vi "Engine Simulation 8 cylinder FPGA.vi"() -> ()   [LabVIEW 2014]
uses:
  <vilib>/NI/Engine Simulation Toolkit (EST)/Version Token.ctl
  <vilib>/NI/Engine Simulation Toolkit (EST)/APU/Settings.ctl
  <vilib>/NI/Engine Simulation Toolkit (EST)/APU/Input.ctl
  <vilib>/NI/Engine Simulation Toolkit (EST)/APU/Output.ctl
  <vilib>/NI/Engine Simulation Toolkit (EST)/Analog Replay/Settings.ctl
  <vilib>/NI/Engine Simulation Toolkit (EST)/Analog Replay/Input.ctl
  <vilib>/NI/Engine Simulation Toolkit (EST)/Analog Replay/Load Input.ctl
  <vilib>/NI/Engine Simulation Toolkit (EST)/Digital Pattern Generation/Load Input.ctl
  <vilib>/NI/Engine Simulation Toolkit (EST)/Digital Pattern Generation/Settings.ctl
  <vilib>/NI/Engine Simulation Toolkit (EST)/Digital Pattern Generation/Input.ctl
  <vilib>/NI/Engine Simulation Toolkit (EST)/ECU Event/Timing/Measure Output.ctl
  <vilib>/NI/Engine Simulation Toolkit (EST)/ECU Event/Timing/Measure Settings.ctl
  <vilib>/NI/Engine Simulation Toolkit (EST)/ECU Event/Timing/Capture Output.ctl
  <vilib>/NI/Engine Simulation Toolkit (EST)/Knock Sensor/Cylinder Input.ctl
  <vilib>/NI/Engine Simulation Toolkit (EST)/Knock Sensor/Cylinder Settings.ctl
  <vilib>/NI/Engine Simulation Toolkit (EST)/Knock Sensor/Generate Input.ctl
  <vilib>/NI/Engine Simulation Toolkit (EST)/Knock Sensor/Generate Settings.ctl
  <vilib>/NI/Engine Simulation Toolkit (EST)/Directional Speed/Load Input.ctl
  <vilib>/NI/Engine Simulation Toolkit (EST)/Directional Speed/Settings.ctl
  <vilib>/NI/Engine Simulation Toolkit (EST)/Directional Speed/Input.ctl
  <vilib>/NI/Engine Simulation Toolkit (EST)/APU/Shared Settings.ctl
  <vilib>/Platform/TimedLoop/XDataNode/timing_clust.ctl
  <vilib>/Platform/TimedLoop/XDataNode/nitl_modes.ctl
  <vilib>/Platform/TimedLoop/XDataNode/wakeup.ctl
  <vilib>/NI/Engine Simulation Toolkit (EST)/ECU Event/Timing/Capture Settings.ctl
  <vilib>/rvi/Emulation/niFpgaGetClockAttributes.vi
  <vilib>/rvi/Emulation/niFpgaSctlEmulationGetInTimedLoop.vi
  <vilib>/rvi/Emulation/niFpgaEmulationReportErrorSimple.vi
  <vilib>/rvi/Emulation/niFpgaCriticalErrorInLSC.vi
  <vilib>/rvi/Emulation/niFpgaProcessEmulError.vi
  <vilib>/rvi/eio/common/nirviEmuTemplateMethod_errors.vi
  <vilib>/rvi/DataTransferAndStorage/Container/Common/niFpgaContainerGetUniqueNameForEmu.vi
  <vilib>/rvi/DataTransferAndStorage/Container/Common/niFpgaContainerSetEmuInfo.vi
  <vilib>/rvi/eio/common/nirviEmuReportErrorAndStop.vi
  <vilib>/NI/Engine Simulation Toolkit (EST)/ECU Event/Timing/Measure Events (40MHz).vi
  <vilib>/Platform/TimedLoop/XDataNode/XDataNode.xnode
  <vilib>/eio/EIONode/EIONode.xnode
  <vilib>/rvi/LocalResourceManager/LocalResourceManager.xnode
  <vilib>/Platform/TimedLoop/XDataNode/XDNodeRunTimeDep.lvlib
  <userlib>/_NI VeriStand FPGA Support/NI VeriStand FPGA Clock Support/NI_VS FPGA Clock Support.lvlib
  <vilib>/NI Veristand/FPGA/NI_VS FPGA Support.lvlib
  <vilib>/NI/Engine Simulation Toolkit (EST)/APU/APU.lvlib
  <vilib>/NI/Engine Simulation Toolkit (EST)/Analog Replay/Analog Replay.lvlib
  <vilib>/NI/Engine Simulation Toolkit (EST)/Digital Pattern Generation/Digital Pattern Generation.lvlib
  <vilib>/NI/Engine Simulation Toolkit (EST)/ECU Event/Timing/ECU Event Timing.lvlib
  <vilib>/NI/Engine Simulation Toolkit (EST)/Knock Sensor/Knock Sensor.lvlib
  <vilib>/NI/Engine Simulation Toolkit (EST)/Directional Speed/Directional Speed.lvlib
  <vilib>/NI/Engine Simulation Toolkit (EST)/Engine Simulation Toolkit.lvlib
panel:
  in  "Tab Control":T1(tab)
  in  "Start":bool
  in  "Loop Rate (usec)":u32
  in  "Write to  RTSI":bool
  in  "Use External Timing":bool
  in  "Generate IRQ":bool
  in  "shared settings.apu 1":T2 {"start" format="%#.15g"}
  in  "go.apu 1":bool
  in  "settings.apu 1":T3 caption="settings"
  out "output.apu 1":T4 caption="output"
  in  "input.apu 1":T5={"desired speed"=0.0, "reset"=TRUE} caption="input"
  in  "est.version":T6
  in  "Spark Tics to Filter":fxp<+,11,11>=350.0
  out "status.Event Spark 6":T7
  out "status.Event Spark 5":T7
  out "status.Event Spark 4":T7
  out "status.Event Spark 3":T7
  out "status.Event Spark 2":T7
  out "status.Event Spark 1":T7
  in  "settings.Event Spark 6":T8
  in  "settings.Event Spark 5":T8
  in  "settings.Event Spark 4":T8
  in  "settings.Event Spark 3":T8
  in  "settings.Event Spark 2":T8
  in  "settings.Event Spark 1":T8
  out "capture.Event Spark 6.Event 1":T9
  out "capture.Event Spark 5.Event 1":T9
  out "capture.Event Spark 4.Event 1":T9
  out "capture.Event Spark 3.Event 1":T9
  out "capture.Event Spark 2.Event 1":T9
  out "capture.Event Spark 1.Event 1":T9
  out "status.Event Spark 7":T7
  in  "settings.Event Spark 7":T8
  out "capture.Event Spark 7.Event 1":T9
  out "status.Event Spark 8":T7
  in  "settings.Event Spark 8":T8
  out "capture.Event Spark 8.Event 1":T9
  in  "Inj Tics to Filter":fxp<+,11,11>=100.0
  out "status.Event Inj 1":T7
  in  "settings.Event Inj 1":T8
  out "capture.Event Inj 1.Event 1":T9
  out "capture.Event Inj 1.Event 2":T9
  out "capture.Event Inj 1.Event 3":T9
  out "capture.Event Inj 1.Event 4":T9
  out "capture.Event Inj 1.Event 5":T9
  out "capture.Event Inj 2.Event 4":T9
  out "capture.Event Inj 2.Event 3":T9
  out "capture.Event Inj 2.Event 2":T9
  out "status.Event Inj 2":T7
  in  "settings.Event Inj 2":T8
  out "capture.Event Inj 2.Event 1":T9
  out "capture.Event Inj 2.Event 5":T9
  out "capture.Event Inj 3.Event 5":T9
  out "capture.Event Inj 3.Event 4":T9
  out "capture.Event Inj 3.Event 3":T9
  out "capture.Event Inj 3.Event 2":T9
  out "status.Event Inj 3":T7
  in  "settings.Event Inj 3":T8
  out "capture.Event Inj 3.Event 1":T9
  out "capture.Event Inj 4.Event 3":T9
  out "capture.Event Inj 4.Event 2":T9
  out "status.Event Inj 4":T7
  in  "settings.Event Inj 4":T8
  out "capture.Event Inj 4.Event 1":T9
  out "capture.Event Inj 4.Event 4":T9
  out "capture.Event Inj 4.Event 5":T9
  in  "settings.Event Inj 7":T8
  in  "settings.Event Inj 6":T8
  in  "settings.Event Inj 8":T8
  in  "settings.Event Inj 5":T8
  out "status.Event Inj 5":T7
  out "capture.Event Inj 5.Event 1":T9
  out "capture.Event Inj 5.Event 5":T9
  out "status.Event Inj 8":T7
  out "capture.Event Inj 8.Event 5":T9
  out "capture.Event Inj 6.Event 3":T9
  out "capture.Event Inj 6.Event 2":T9
  out "status.Event Inj 7":T7
  out "capture.Event Inj 8.Event 4":T9
  out "capture.Event Inj 8.Event 3":T9
  out "capture.Event Inj 8.Event 2":T9
  out "capture.Event Inj 8.Event 1":T9
  out "status.Event Inj 6":T7
  out "capture.Event Inj 6.Event 1":T9
  out "capture.Event Inj 5.Event 4":T9
  out "capture.Event Inj 5.Event 3":T9
  out "capture.Event Inj 5.Event 2":T9
  out "capture.Event Inj 6.Event 5":T9
  out "capture.Event Inj 6.Event 4":T9
  out "capture.Event Inj 7.Event 5":T9
  out "capture.Event Inj 7.Event 4":T9
  out "capture.Event Inj 7.Event 3":T9
  out "capture.Event Inj 7.Event 2":T9
  out "capture.Event Inj 7.Event 1":T9
  in  "load input.Dir Speed 1":T10
  in  "settings.Dir Speed 2":T11
  in  "input.Dir Speed 2":T12
  in  "settings.Dir Speed 1":T11
  in  "input.Dir Speed 1":T12
  in  "load input.Dir Speed 2":T10
  in  "load input.Crank":T13
  in  "settings.Aux Pattern":T14
  in  "input.Aux Pattern":T15
  in  "settings.Cam 2":T14
  in  "input.Cam 2":T15
  in  "settings.Cam 1":T14
  in  "input.Cam 1":T15
  in  "settings.Crank":T14
  in  "input.Crank":T15
  in  "load input.Cam 1":T13
  in  "load input.Cam 2":T13
  in  "load input.Aux Pattern":T13
  in  "settings.VR 1":T16 caption="settings"
  in  "settings.VR 2":T16 caption="settings"
  in  "input.VR 2":T17 caption="input"
  in  "input.VR 1":T17 caption="input"
  in  "load input.VR 1":T18={"Data"=[0, 0, 0, 0, 0, 0, 0, 0, 0, 0, 0, 0, 0, 0, 0, 0], "LoadOffset"=0, "Done"=FALSE} caption="input"
  in  "load input.VR 2":T18={"Data"=[0, 0, 0, 0, 0, 0, 0, 0, 0, 0, 0, 0, 0, 0, 0, 0], "LoadOffset"=0, "Done"=FALSE} caption="input"
  in  "input.Knock 1.Cylinder 4":T19={"probability compare"=65535, "high freq scaler"=0.0, "trigger position"=0}
  in  "input.Knock 1.Cylinder 3":T19={"probability compare"=65535, "high freq scaler"=0.0, "trigger position"=0}
  in  "input.Knock 1.Cylinder 2":T19={"probability compare"=65535, "high freq scaler"=0.0, "trigger position"=0}
  in  "input.Knock 1.Cylinder 1":T19={"probability compare"=65535, "high freq scaler"=0.0, "trigger position"=0}
  in  "settings.Knock 1.Cylinder 4":T20
  in  "settings.Knock 1.Cylinder 3":T20
  in  "settings.Knock 1.Cylinder 2":T20
  in  "settings.Knock 1.Cylinder 1":T20
  in  "input.Knock 1":T21
  in  "settings.Knock 1":T22
  in  "input.Knock 1.Cylinder 5":T19={"probability compare"=65535, "high freq scaler"=0.0, "trigger position"=0}
  in  "settings.Knock 1.Cylinder 5":T20
  in  "input.Knock 1.Cylinder 8":T19={"probability compare"=65535, "high freq scaler"=0.0, "trigger position"=0}
  in  "settings.Knock 1.Cylinder 8":T20
  in  "input.Knock 1.Cylinder 7":T19={"probability compare"=65535, "high freq scaler"=0.0, "trigger position"=0}
  in  "settings.Knock 1.Cylinder 7":T20
  in  "input.Knock 1.Cylinder 6":T19={"probability compare"=65535, "high freq scaler"=0.0, "trigger position"=0}
  in  "settings.Knock 1.Cylinder 6":T20
  in  "input.Knock 2.Cylinder 4":T19
  in  "input.Knock 2.Cylinder 3":T19
  in  "input.Knock 2.Cylinder 2":T19
  in  "input.Knock 2.Cylinder 1":T19
  in  "settings.Knock 2.Cylinder 4":T20
  in  "settings.Knock 2.Cylinder 3":T20
  in  "settings.Knock 2.Cylinder 2":T20
  in  "settings.Knock 2.Cylinder 1":T20
  in  "input.Knock 2.Cylinder 7":T19
  in  "settings.Knock 2.Cylinder 7":T20
  in  "input.Knock 2.Cylinder 5":T19
  in  "settings.Knock 2.Cylinder 5":T20
  in  "input.Knock 2.Cylinder 8":T19
  in  "settings.Knock 2.Cylinder 8":T20
  in  "input.Knock 2.Cylinder 6":T19
  in  "settings.Knock 2.Cylinder 6":T20
  in  "input.Knock 2":T21
  in  "settings.Knock 2":T22
  in  "PulseGen Packets 0-7":u64[](array[numeric])=[0, 0, 0, 0, 0, 0, 0, 0]
  in  "PWM.In.7.Timeout":u32=40000
  in  "PWM.In.6.Timeout":u32=40000
  in  "PWM.In.5.Timeout":u32=40000
  in  "PWM.In.4.Timeout":u32=40000
  in  "PWM.In.3.Timeout":u32=40000
  in  "PWM.In.2.Timeout":u32=40000
  in  "PWM.In.1.Timeout":u32=40000
  in  "PWM.In.0.Timeout":u32=40000
  out "PulseMeas Packets 0-7":u64[](array[numeric])
  in  "PWM.In.15.Timeout":u32=40000
  in  "PWM.In.14.Timeout":u32=40000
  in  "PWM.In.13.Timeout":u32=40000
  in  "PWM.In.12.Timeout":u32=40000
  in  "PWM.In.11.Timeout":u32=40000
  in  "PWM.In.10.Timeout":u32=40000
  in  "PWM.In.9.Timeout":u32=40000
  in  "PWM.In.8.Timeout":u32=40000
  out "PulseMeas Packets 2 8-15":u64[](array[numeric])
  in  "PulseGen Packets 8-15":u64[](array[numeric])=[0, 0, 0, 0, 0, 0, 0, 0]
  in  "PulseMeas 7 Timeout":u32=40000
  in  "PulseMeas 6 Timeout":u32=40000
  in  "PulseMeas 5 Timeout":u32=40000
  in  "PulseMeas 4 Timeout":u32=40000
  in  "PulseMeas 3 Timeout":u32=40000
  in  "PulseMeas 2 Timeout":u32=40000
  in  "PulseMeas 1 Timeout":u32=40000
  in  "PulseMeas 0 Timeout":u32=40000
  out "PulseMeas Packets 8-15":u64[](array[numeric])
  in  "PulseGen Packets":u64[](array[numeric])=[0, 0, 0, 0, 0, 0, 0, 0]
  # "DC"
  # "f"
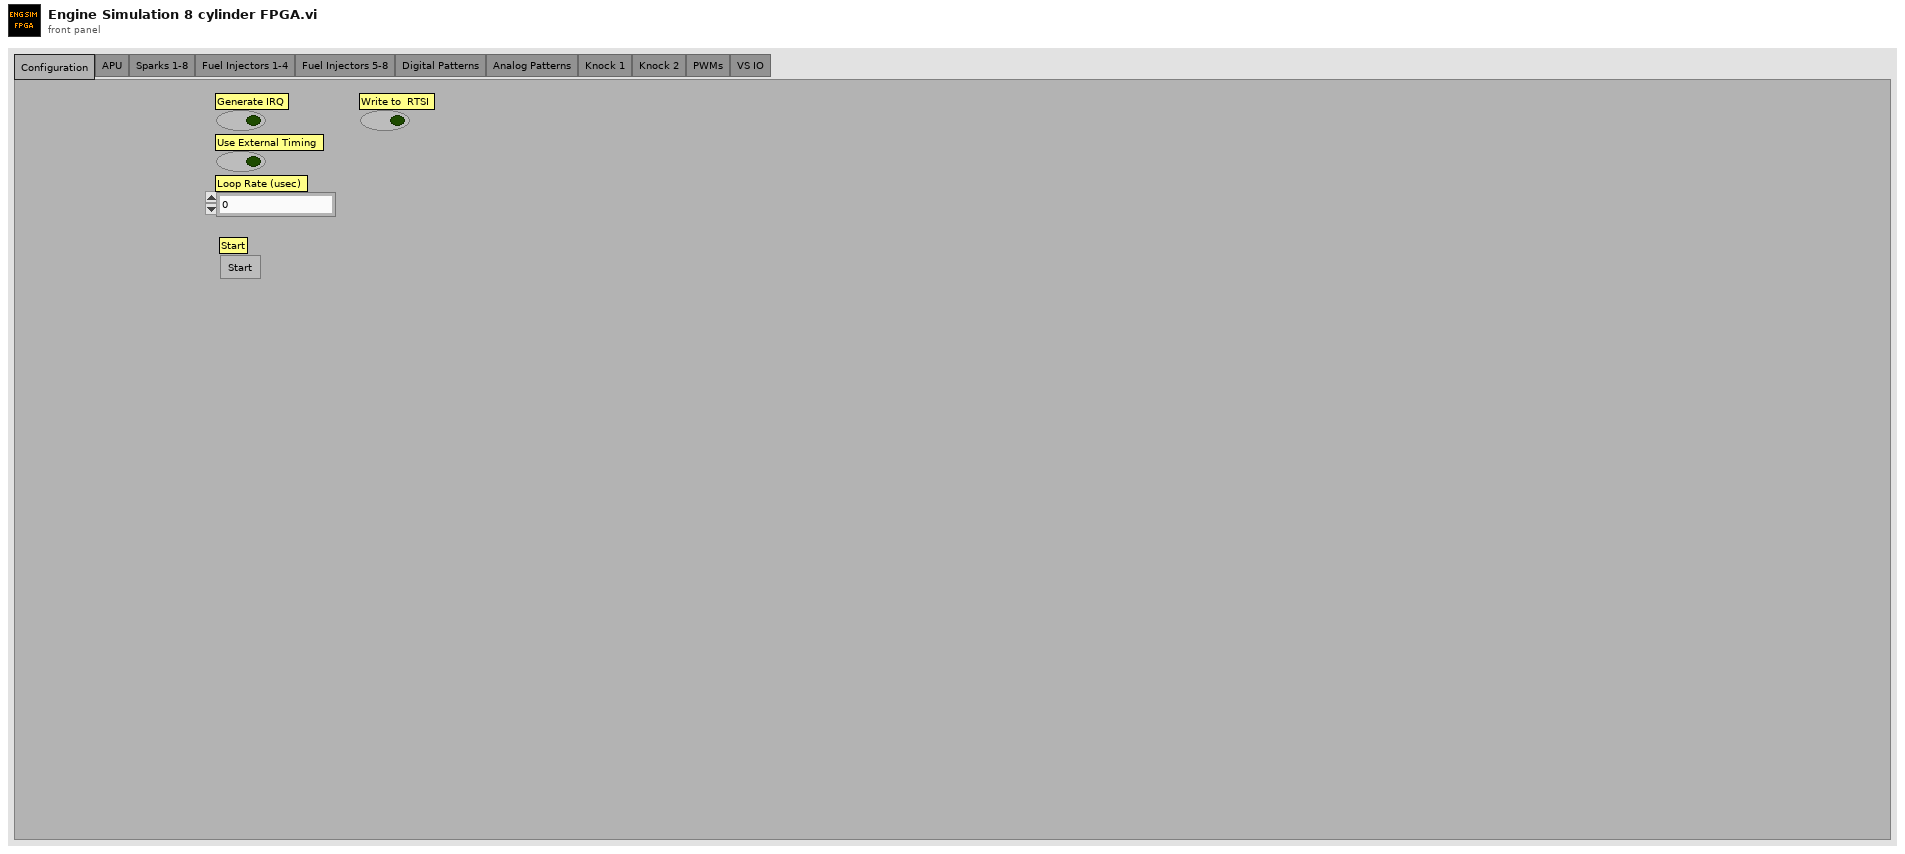
[diagram p1: front panel]
types:
  T1 = enum32{"Configuration", "APU", "Sparks 1-8", "Fuel Injectors 1-4", "Fuel Injectors 5-8", "Digital Patterns", "Analog Patterns", "Knock 1", "Knock 2", "PWMs", "VS IO"}
  T2 = typedef "Engine Simulation Toolkit.lvlib/APU.lvlib/Shared Settings.ctl" = cluster{"start":fxp<+,17,17>, "stuck limit":fxp<+,18,18>}
  T3 = typedef "Engine Simulation Toolkit.lvlib/APU.lvlib/Settings.ctl" = cluster{"acceleration":fxp<+,18,-20>, "enable accel":bool}
  T4 = typedef "Engine Simulation Toolkit.lvlib/APU.lvlib/Output.ctl" = cluster{"crank":u16, "cycle":u16, "actual speed":fxp<+/-,23,2>}
  T5 = typedef "Engine Simulation Toolkit.lvlib/APU.lvlib/Input.ctl" = cluster{"desired speed":fxp<+/-,23,2>, "reset":bool}
  T6 = typedef "Engine Simulation Toolkit.lvlib/Version Token.ctl" = cluster{"1.3.0":bool}
  T7 = typedef "Engine Simulation Toolkit.lvlib/ECU Event Timing.lvlib/Measure Output.ctl" = cluster{"stuck active":bool, "window all active":bool, "window orphan start":bool, "window orphan end":bool}
  T8 = typedef "Engine Simulation Toolkit.lvlib/ECU Event Timing.lvlib/Measure Settings.ctl" = cluster{"max":u16, "min":u16, "active high":bool, "wrap":bool}
  T9 = typedef "Engine Simulation Toolkit.lvlib/ECU Event Timing.lvlib/Capture Output.ctl" = cluster{"Start":u16, "End":u16, "Duration (tics)":fxp<+,18,18>, "Event present":bool}
  T10 = typedef "Engine Simulation Toolkit.lvlib/Directional Speed.lvlib/Load Input.ctl" = cluster{"address":fxp<+,10,10>, "done":bool, "angle":u16}
  T11 = typedef "Engine Simulation Toolkit.lvlib/Directional Speed.lvlib/Settings.ctl" = cluster{"Upper Value":u16, "Lower Value":u16, "Upper Index":fxp<+,10,10>, "Lower Index":fxp<+,10,10>, "Enabled":bool}
  T12 = typedef "Engine Simulation Toolkit.lvlib/Directional Speed.lvlib/Input.ctl" = cluster{"td (tics)":u16, "tf (tics)":u16, "tr (tics)":u16}
  T13 = typedef "Engine Simulation Toolkit.lvlib/Digital Pattern Generation.lvlib/Load Input.ctl" = cluster{"address":fxp<+,11,11>, "done":bool, "angle":u16}
  T14 = typedef "Engine Simulation Toolkit.lvlib/Digital Pattern Generation.lvlib/Settings.ctl" = cluster{"edge 1":u16, "edge 2":u16, "cycle angle":bool, "enabled":bool, "first falling":bool, "fault":bool, "fault wrap":bool, "fault value":bool, "fault count":fxp<+,4,4>, "use fault count":bool}
  T15 = typedef "Engine Simulation Toolkit.lvlib/Digital Pattern Generation.lvlib/Input.ctl" = cluster{"Offset":i16}
  T16 = typedef "Engine Simulation Toolkit.lvlib/Analog Replay.lvlib/Settings.ctl" = cluster{"ReverseNegate":bool, "CycleAngle":bool, "SpeedThreshold":fxp<+/-,23,2>, "AOBelowThreshold":i16}
  T17 = typedef "Engine Simulation Toolkit.lvlib/Analog Replay.lvlib/Input.ctl" = cluster{"Offset":i16, "VScaleSlope":fxp<+,18,6>, "VScaleIntercept":fxp<+/-,18,3>}
  T18 = typedef "Engine Simulation Toolkit.lvlib/Analog Replay.lvlib/Load Input.ctl" = cluster{"Data":i16[], "LoadOffset":u16, "Done":bool}
  T19 = typedef "Engine Simulation Toolkit.lvlib/Knock Sensor.lvlib/Cylinder Input.ctl" = cluster{"probability compare":u16, "high freq scaler":fxp<+,10,0>, "trigger position":u16}
  T20 = typedef "Engine Simulation Toolkit.lvlib/Knock Sensor.lvlib/Cylinder Settings.ctl" = cluster{"seed":u16, "reset":bool}
  T21 = typedef "Engine Simulation Toolkit.lvlib/Knock Sensor.lvlib/Generate Input.ctl" = cluster{"low freq scaler":fxp<+,10,0>}
  T22 = typedef "Engine Simulation Toolkit.lvlib/Knock Sensor.lvlib/Generate Settings.ctl" = cluster{"low freq (periods/tick)":fxp<+,32,0>, "high freq (periods/tick)":fxp<+,32,0>, "duration (1.25MHz tics)":fxp<+,18,18>, "low freq speed slope":fxp<+,16,-3>, "low freq speed intercept":fxp<+,10,-10>, "low freq by speed":bool}
  T23 = typedef "XDNodeRunTimeDep.lvlib/timing_clust.ctl" = cluster{"Expected End [f-1]":u64, "Actual End [f-1]":u64, "Finished Late? [f-1]":bool, "Expected End [i-1]":u64, "Actual End [i-1]":u64, "Finished Late? [i-1]":bool, "Expected Start [i]":u64, "Actual Start [i]":u64, "Expected Start [f]":u64, "Actual Start [f]":u64, "Source Name":string, "Structure Name":string, "Period":i64, "Deadline":i64, "Offset":i64, "Start":i64, "Priority":i32, "Timeout":i32, "Mode":T24, "Wakeup Reason":T25, "Error":errorcluster, "Source Type":string, "Secondary Source Type":string, "Global End Time":u64, "Global Start Time":u64, "Frame Duration":u64, "Iteration Duration":u64, "Assigned CPU":i32, "I/O Scan Engine Mode":u32}
  T24 = typedef "XDNodeRunTimeDep.lvlib/nitl_modes.ctl" = enum32{"No Change", "Process missed periods, maintain original phase", "Discard missed periods, maintain original phase", "Process missed periods, ignore original phase", "Discard missed periods, ignore original phase"}
  T25 = typedef "XDNodeRunTimeDep.lvlib/wakeup.ctl" = enum32{"Normal", "Aborted", "Asynchronous wakeup", "Timing source error", "Timed loop error", "Timeout"}
  T26 = cluster{"DO0":refnum<k21>, "DO1":refnum<k21>, "DO2":refnum<k21>, "DO3":refnum<k21>, "DO4":refnum<k21>, "DO5":refnum<k21>, "DO6":refnum<k21>, "DO7":refnum<k21>}
  T27 = cluster{"DI0":refnum<k21>, "DI1":refnum<k21>, "DI2":refnum<k21>, "DI3":refnum<k21>, "DI4":refnum<k21>, "DI5":refnum<k21>, "DI6":refnum<k21>, "DI7":refnum<k21>}
  T28 = typedef "Engine Simulation Toolkit.lvlib/Digital Pattern Generation.lvlib/Load Data.ctl" = cluster{"max address":fxp<+,11,11>, "memory":refnum<k21>}
  T29 = typedef "Engine Simulation Toolkit.lvlib/APU.lvlib/Register Bus.ctl" = cluster{"Speed":refnum<k21>, "Crank Angle":refnum<k21>, "Cycle Angle":refnum<k21>, "Crank Count":refnum<k21>, "Cycle Count":refnum<k21>, "1.25 MHz Counter":refnum<k21>, "Crank Rollover":refnum<k21>, "Cycle Rollover":refnum<k21>, "shared settings":T2}
  T30 = typedef "Engine Simulation Toolkit.lvlib/Directional Speed.lvlib/Load Data.ctl" = cluster{"max address":fxp<+,10,10>, "Memory":refnum<k21>}
  T31 = typedef "Engine Simulation Toolkit.lvlib/Knock Sensor.lvlib/Triggered Cylinder Data.ctl" = cluster{"trigger knock":bool, "high freq scaler":fxp<+,10,0>}
  T32 = typedef "Engine Simulation Toolkit.lvlib/ECU Event Timing.lvlib/Capture Settings.ctl" = u8
  T33 = typedef "Engine Simulation Toolkit.lvlib/ECU Event Timing.lvlib/Measured Data.ctl" = cluster{"start":u16, "end":u16, "duration (tics)":fxp<+,18,18>, "window end":bool, "window begin":bool, "pulse end":bool, "pulse #":u8}
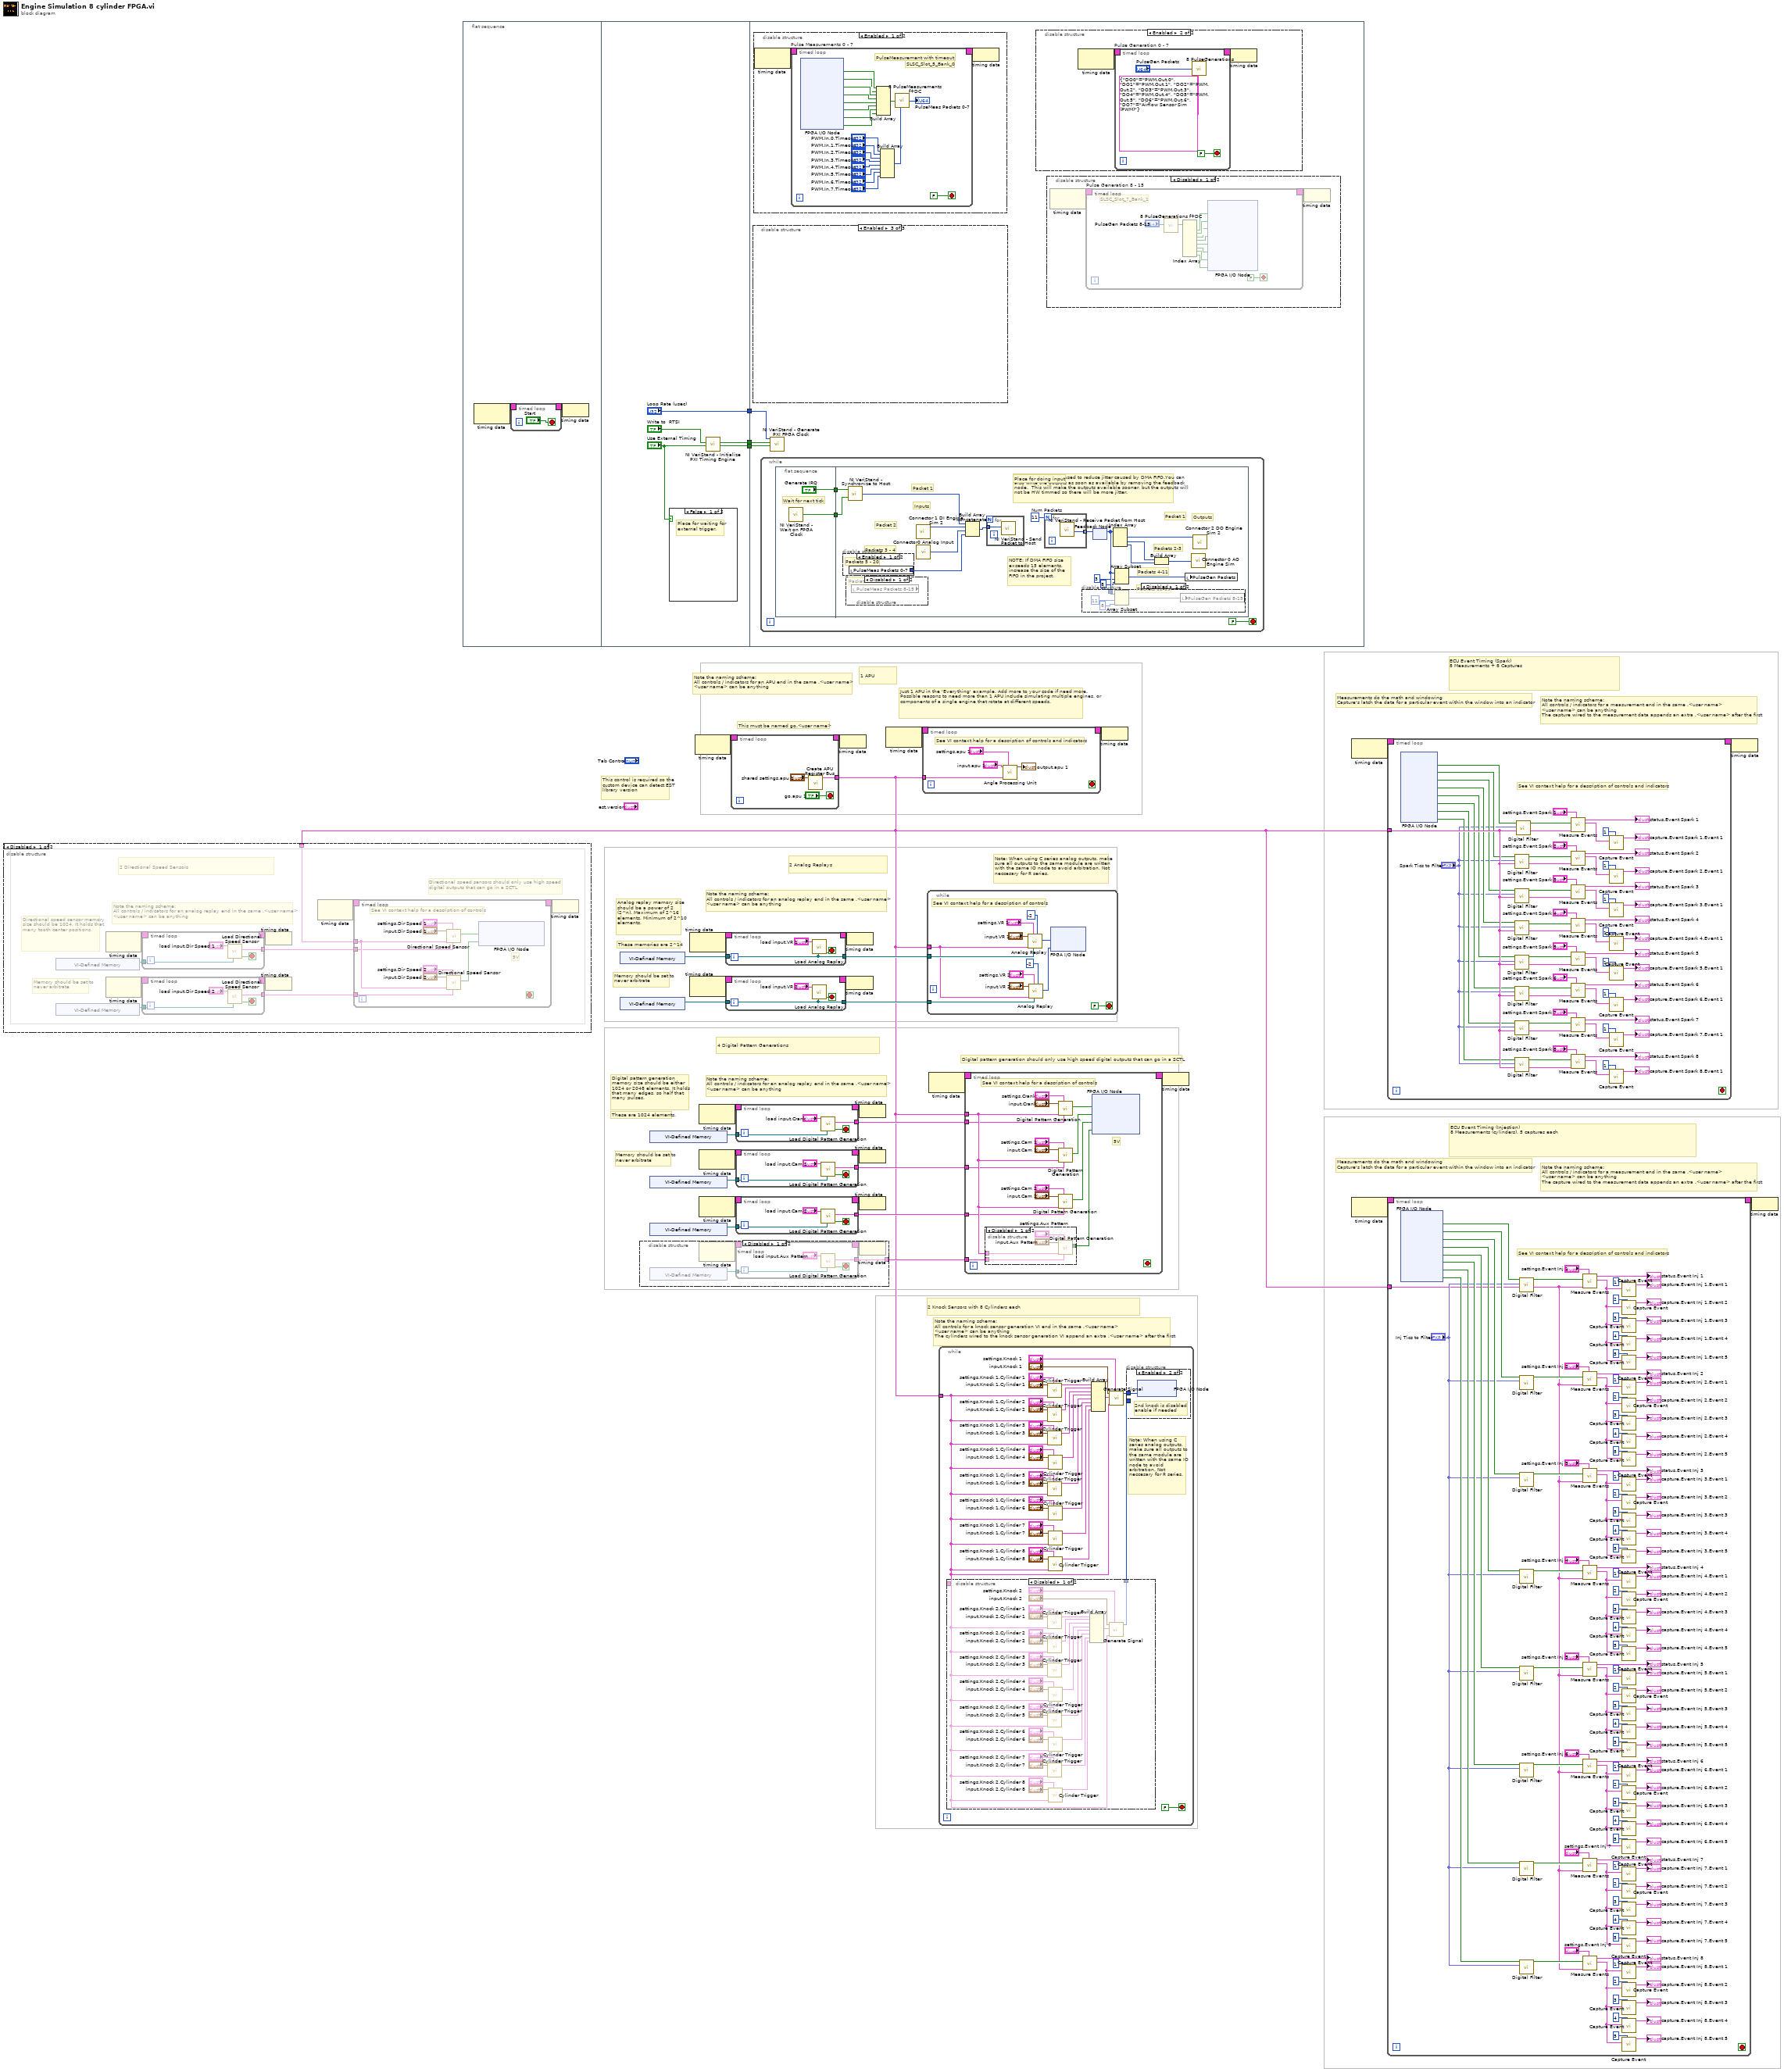
[diagram p0: block diagram]
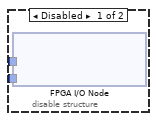
[diagram p5: hidden frame]
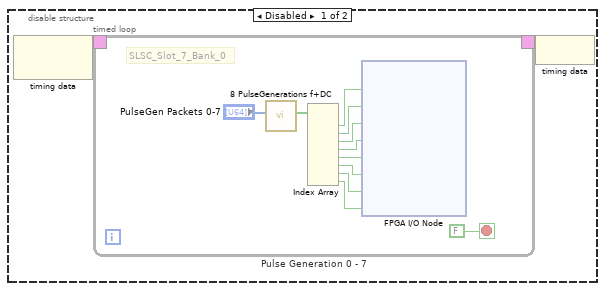
[diagram p9: hidden frame]
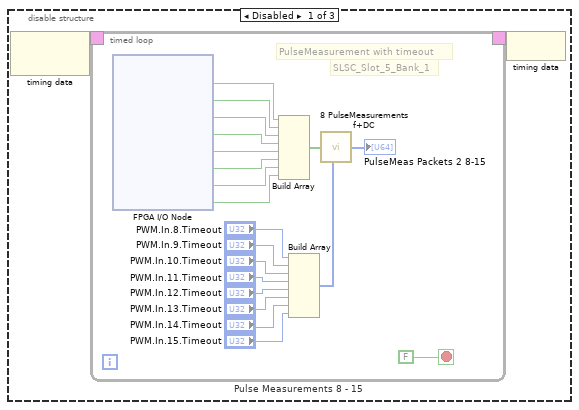
[diagram p11: hidden frame]
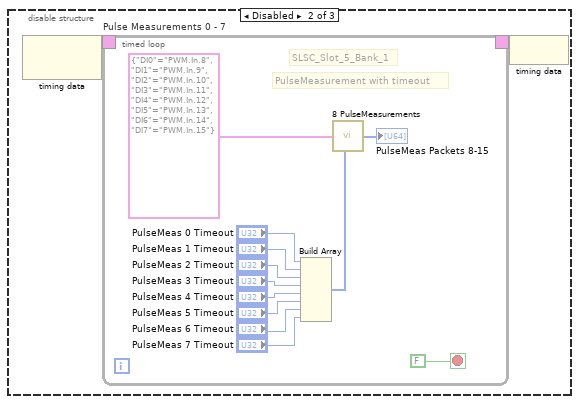
[diagram p12: hidden frame]
diagram:
  # "This must be named go.<user name>"
  # "Memory should be set to never arbitrate"
  # "Memory should be set to never arbitrate"
  # "Note the naming scheme: \nAll controls for a knock sensor generation VI end in the same .<user name>\n<user name> can be anything\nThe cylinders wired to the knock sensor generation VI append an extra .<user name> after the first"
  # "2 Knock Sensors with 8 Cylinders each"
  # "Measurements do the math and windowing\nCapture's latch the data for a particular event within the window into an indicator"
  # "ECU Event Timing (Injection)\n8 Measurements (cylinders), 5 captures each"
  # "Note the naming scheme: \nAll controls / indicators for a measurement end in the same .<user name>\n<user name> can be anything\nThe capture wired to the measurement data appends an extra .<user name> after the first"
  # "Measurements do the math and windowing\nCapture's latch the data for a particular event within the window into an indicator"
  # "ECU Event Timing (Spark)\n8 Measurements + 8 Captures"
  # "Note the naming scheme: \nAll controls / indicators for a measurement end in the same .<user name>\n<user name> can be anything\nThe capture wired to the measurement data appends an extra .<user name> after the first"
  # "Digital pattern generation should only use high speed digital outputs that can go in a SCTL"
  # "4 Digital Pattern Generations"
  # "Note the naming scheme: \nAll controls / indicators for an analog replay end in the same .<user name>\n<user name> can be anything"
  # "These are 1024 elements."
  # "Digital pattern generation memory size should be either 1024 or 2048 elements. It holds that many edges, so half that many pulses."
  # "Note: When using C series analog outputs, make sure all outputs to the same module are written with the same IO node to avoid arbitration. Not neccesary for R series."
  # "2 Analog Replays"
  # "1 APU"
  # "These memories are 2^14"
  # "Note the naming scheme: \nAll controls / indicators for an APU end in the same .<user name>\n<user name> can be anything"
  # "Note the naming scheme: \nAll controls / indicators for an analog replay end in the same .<user name>\n<user name> can be anything"
  # "Analog replay memory size should be a power of 2 (2^n). Maximum of 2^16 elements. Minimum of 2^10 elements."
  # "Just 1 APU in the 'Everything' example. Add more to your code if need more. Possible reasons to need more than 1 APU include simulating multiple engines, or components of a single engine that rotate at different speeds."
  # "This control is required so the custom device can detect EST library version"
  n1 = flat-sequence {
    tunnel: [w44] -> w35
    tunnel: ["Loop Rate (usec)"] -> w34
    tunnel: [w43] -> w33
    tunnel: w35 -> [w50]
    tunnel: w34 -> [w49]
    tunnel: w33 -> [w48]
    frame #0 {
      n2 = node-c288() -> (w37:T23)  [unwired: 1 out]
      n3 = timed-loop {
        timing: w37 -> [_]
        timing-out: [_] -> w36
        stop <- "Start" stop-if-true
      }
      n4 = node-c288(w36) -> ()
    }
    frame #1 {
      n5 = case shown="False" "Use External Timing" {
        frame False {
          # "Place for waiting for external trigger."
        }
        frame True {
          # "Do not wait on trigger when externally timed."
        }
      }
      n6 = call <userlib>:"NI VeriStand - Initialize PXI Timing Engine.vi"("Use External Timing In"="Use External Timing", "Write to  RTSI In"="Write to  RTSI") -> ("Use External Timing Out"=w44:bool, "Write to  RTSI Out"=w43:bool)  [unwired: 8 in]
    }
    frame #2 {
      n7 = disable-structure shown="Enabled" {
        frame Disabled {
          n8 = node-c288() -> (w121:T23)  [unwired: 1 out]
          n9 = timed-loop "Pulse Measurements 8 - 15" {
            timing: w121 -> [_]
            timing-out: [_] -> w120
            stop <- FALSE stop-if-true
            # "SLSC_Slot_5_Bank_1"
            # "PulseMeasurement with timeout"
            n10 = xnode "FPGA I/O Node"() -> ("PWM.In.8"=w124:bool, "PWM.In.9"=w125:bool, "PWM.In.10"=w126:bool, "PWM.In.11"=w127:bool, "PWM.In.12"=w128:bool, "PWM.In.13"=w129:bool, "PWM.In.14"=w130:bool, "PWM.In.15"=w123:bool)  [unwired: 8 in, 8 out]
            n11 = Build Array(w124, w125, w126, w127, w128, w129, w130, w123) -> (w122:bool[])
            n12 = Build Array("PWM.In.8.Timeout", "PWM.In.9.Timeout", "PWM.In.10.Timeout", "PWM.In.11.Timeout", "PWM.In.12.Timeout", "PWM.In.13.Timeout", "PWM.In.14.Timeout", "PWM.In.15.Timeout") -> (w140:u32[])
            n13 = call "8 PulseMeasurements f+DC.vi"("8 PulseMeas Chs"=w122, "PulseMeas Timeouts"=w140) -> ("PulseMeas Packets DC-f"=→"PulseMeas Packets 2 8-15":u64[])  [unwired: 7 in]
          }
          n14 = node-c288(w120) -> ()
        }
        frame Disabled {
          n15 = node-c288() -> (w147:T23)  [unwired: 1 out]
          n16 = timed-loop "Pulse Measurements 0 - 7" {
            timing: w147 -> [_]
            timing-out: [_] -> w146
            stop <- FALSE stop-if-true
            # "SLSC_Slot_5_Bank_1"
            # "PulseMeasurement with timeout"
            n17 = Build Array("PulseMeas 0 Timeout", "PulseMeas 1 Timeout", "PulseMeas 2 Timeout", "PulseMeas 3 Timeout", "PulseMeas 4 Timeout", "PulseMeas 5 Timeout", "PulseMeas 6 Timeout", "PulseMeas 7 Timeout") -> (w158:u32[])
            n18 = call <userlib>:"8 PulseMeasurements.vi"("8 PulseMeas Chs"=T27 {"DI0"="PWM.In.8", "DI1"="PWM.In.9", "DI2"="PWM.In.10", "DI3"="PWM.In.11", "DI4"="PWM.In.12", "DI5"="PWM.In.13", "DI6"="PWM.In.14", "DI7"="PWM.In.15"}, "PulseMeas Timeouts"=w158) -> ("PulseMeas Packets"=→"PulseMeas Packets 8-15":u64[])  [unwired: 7 in]
          }
          n19 = node-c288(w146) -> ()
        }
        frame Enabled {
        }
      }
      n20 = disable-structure shown="Enabled" {
        frame Enabled {
          n21 = node-c288() -> (w52:T23)  [unwired: 1 out]
          n22 = timed-loop "Pulse Measurements 0 - 7" {
            timing: w52 -> [_]
            timing-out: [_] -> w51
            stop <- FALSE stop-if-true
            # "SLSC_Slot_5_Bank_0"
            # "PulseMeasurement with timeout"
            n23 = xnode "FPGA I/O Node"() -> ("PWM.In.0"=w55:bool, "PWM.In.1"=w56:bool, "PWM.In.2"=w57:bool, "PWM.In.3"=w58:bool, "PWM.In.4"=w59:bool, "PWM.In.5"=w60:bool, "PWM.In.6"=w61:bool, "PWM.In.7"=w54:bool)  [unwired: 8 in, 8 out]
            n24 = Build Array(w55, w56, w57, w58, w59, w60, w61, w54) -> (w53:bool[])
            n25 = Build Array("PWM.In.0.Timeout", "PWM.In.1.Timeout", "PWM.In.2.Timeout", "PWM.In.3.Timeout", "PWM.In.4.Timeout", "PWM.In.5.Timeout", "PWM.In.6.Timeout", "PWM.In.7.Timeout") -> (w71:u32[])
            n26 = call "8 PulseMeasurements f+DC.vi"("8 PulseMeas Chs"=w53, "PulseMeas Timeouts"=w71) -> ("PulseMeas Packets DC-f"=→"PulseMeas Packets 0-7":u64[])  [unwired: 7 in]
          }
          n27 = node-c288(w51) -> ()
        }
        frame Disabled {
        }
      }
      n28 = while {
        stop <- FALSE stop-if-true
        n29 = flat-sequence {
          tunnel: ["Generate IRQ"] -> w165
          tunnel: [w167] -> w164
          tunnel: w165 -> [w185]
          tunnel: w164 -> [w184]
          frame #0 {
            # "Wait for next tick"
            n30 = call <userlib>:"NI VeriStand - Wait on FPGA Clock.vi"() -> ("Clock Ticked"=w167:bool)
          }
          frame #1 {
            w183 = 11  # Num Packets
            # "Packet 2"
            # "Packets 12-19"
            # "Packets 4-11"
            # "Packets 2-3"
            # "Packet 1"
            # "Packets 3 - 4"
            # "Inputs"
            # "Outputs"
            # "Packet 1"
            # "NOTE: If DMA FIFO size exceeds 15 elements, increase the size of the FIFO in the project."
            # "Feedback nodes are used to reduce jitter caused by DMA FIFO.You can also write the outputs as soon as available by removing the feedback node.  This will make the outputs available sooner, but the outputs will not be HW timmed so there will be more jitter."
            # "Place for doing input"
            n31 = disable-structure shown="Enabled" {
              disable-tunnel: [w186 _] -> w169
              frame Enabled {
                # "Packets 5 - 20"
                n32 = local read "PulseMeas Packets 0-7"() -> (w186:u64[])
              }
              frame Disabled {
              }
            }
            n33 = disable-structure shown="Disabled" {
              frame Disabled {
                # "Packets 21 - 28"
                n34 = local read "PulseMeas Packets 8-15"() -> ()  [unwired: 1 out]
              }
              frame Enabled {
              }
            }
            n35 = call <userlib>:"NI VeriStand - Synchronize to Host.vi"("Clock Ticked"=w184, "Generate IRQ"=w185) -> ("Is Late?"=w182:u64)
            n36 = call "Connector 1 DI Engine Sim 2.vi"() -> ("Packet"=w174:u64)  [unwired: 11 in]
            n37 = call <userlib>:"Connector0 Analog Input.vi"() -> ("Packets"=w180:u64[])
            n38 = Build Array (concatenate)(w182, w174, w180, w169) -> (w181:u64[])
            n39 = for {
              tunnel: w181 -> [w191] mode=indexing
              n40 = call <vilib>:"NI VeriStand - Send Packet to Host.vi"("Element"=w191) -> ()  [unwired: 2 in, 9 out]
            }
            n41 = for {
              N: w183 -> [_]
              tunnel: [w192] -> w179 mode=indexing
              n42 = call <vilib>:"NI VeriStand - Receive Packet from Host.vi"() -> ("Element"=w192:u64)  [unwired: 2 in, 9 out]
            }
            n43 = feedback-in #1(w179) -> ()
            n44 = feedback #1() -> (w173:u64[])  [unwired: 1 in]
            n45 = disable-structure shown="Disabled" {
              disable-tunnel: w173 -> [w190 _]
              frame Disabled {
                n46 = Array Subset(array=w190, index=11, length=8) -> (w187:u64[])
                n47 = local write "PulseGen Packets 8-15"(w187) -> ()
              }
              frame Enabled {
              }
            }
            n48 = Index Array(array=w173) -> (element #1=w175:u64, element #2=w178:u64, element #3=w177:u64)  [unwired: 3 in]
            n49 = Array Subset(array=w173, index=3, length=8) -> (w170:u64[])
            n50 = Build Array(w178, w177) -> (w176:u64[])
            n51 = local write "PulseGen Packets"(w170) -> ()
            n52 = call "Connector 0 AO Engine Sim.vi"("Packets"=w176) -> ()
            n53 = call "Connector 2 DO Engine Sim 2.vi"("Packet"=w175) -> ()  [unwired: 11 in]
          }
        }
      }
      n54 = call <userlib>:"NI VeriStand - Generate PXI FPGA Clock.vi"("Use External Timing"=w50, "Write to  RTSI"=w48, "Loop Rate (usec)"=w49) -> ()  [unwired: 9 in]
      n55 = disable-structure shown="Enabled" {
        frame Disabled {
          n56 = node-c288() -> (w78:T23)  [unwired: 1 out]
          n57 = timed-loop "Pulse Generation 0 - 7" {
            timing: w78 -> [_]
            timing-out: [_] -> w77
            stop <- FALSE stop-if-true
            # "SLSC_Slot_7_Bank_0"
            n58 = call "8 PulseGenerations f+DC.vi"("PulseGen Packets"="PulseGen Packets 0-7") -> ("PWMs"=w87:bool[])  [unwired: 8 in]
            n59 = Index Array(array=w87) -> (element #1=w86:bool, element #2=w85:bool, element #3=w84:bool, element #4=w83:bool, element #5=w82:bool, element #6=w81:bool, element #7=w80:bool, element #8=w79:bool)  [unwired: 8 in]
            n60 = xnode "FPGA I/O Node"("PWM.Out.0"=w86, "PWM.Out.1"=w85, "PWM.Out.2"=w84, "PWM.Out.3"=w83, "PWM.Out.4"=w82, "PWM.Out.5"=w81, "PWM.Out.6"=w80, "PWM.Out.7"=w79) -> ()  [unwired: 8 in, 8 out]
          }
          n61 = node-c288(w77) -> ()
        }
        frame Enabled {
          n62 = node-c288() -> (w95:T23)  [unwired: 1 out]
          n63 = timed-loop "Pulse Generation 0 - 7" {
            timing: w95 -> [_]
            timing-out: [_] -> w94
            stop <- FALSE stop-if-true
            n64 = call <userlib>:"8 PulseGenerations.vi"("PulseGen Packets"="PulseGen Packets", "8 PulseGen Chs"=T26 {"DO0"="PWM.Out.0", "DO1"="PWM.Out.1", "DO2"="PWM.Out.2", "DO3"="PWM.Out.3", "DO4"="PWM.Out.4", "DO5"="PWM.Out.5", "DO6"="PWM.Out.6", "DO7"="Airflow Sensor Sim (PWM)"}) -> ()  [unwired: 8 in]
          }
          n65 = node-c288(w94) -> ()
        }
      }
      n66 = disable-structure shown="Disabled" {
        frame Disabled {
          n67 = node-c288() -> (w104:T23)  [unwired: 1 out]
          n68 = timed-loop "Pulse Generation 8 - 15" {
            timing: w104 -> [_]
            timing-out: [_] -> w103
            stop <- FALSE stop-if-true
            # "SLSC_Slot_7_Bank_1"
            n69 = call "8 PulseGenerations f+DC.vi"("PulseGen Packets"="PulseGen Packets 8-15") -> ("PWMs"=w113:bool[])  [unwired: 8 in]
            n70 = Index Array(array=w113) -> (element #1=w112:bool, element #2=w111:bool, element #3=w110:bool, element #4=w109:bool, element #5=w108:bool, element #6=w107:bool, element #7=w106:bool, element #8=w105:bool)  [unwired: 8 in]
            n71 = xnode "FPGA I/O Node"("PWM.Out.8"=w112, "PWM.Out.9"=w111, "PWM.Out.10"=w110, "PWM.Out.11"=w109, "PWM.Out.12"=w108, "PWM.Out.13"=w107, "PWM.Out.14"=w106, "PWM.Out.15"=w105) -> ()  [unwired: 8 in, 8 out]
          }
          n72 = node-c288(w103) -> ()
        }
        frame Enabled {
        }
      }
    }
  }
  n73 = xnode "VI-Defined Memory"() -> ("Memory Out"=w11:refnum<k21>)
  n74 = xnode "VI-Defined Memory"() -> ("Memory Out"=w12:refnum<k21>)
  n75 = disable-structure shown="Disabled" {
    disable-tunnel: [w193 _] -> w4
    frame Disabled {
      n76 = xnode "VI-Defined Memory"() -> ("Memory Out"=w194:refnum<k21>)
      n77 = node-c288() -> (w196:T23)  [unwired: 1 in]
      n78 = timed-loop {
        timing: w196 -> [_]
        timing-out: [_] -> w195
        tunnel: w194 -> [w199]
        tunnel: [w198] -> w193
        stop <- w200 stop-if-true
        n79 = call <vilib>:"Load Digital Pattern Generation.vi"("memory"=w199, "load input.<user name>"="load input.Aux Pattern") -> ("done"=w200:bool, "load data"=w198:T28)  [unwired: 8 in]
      }
      n80 = node-c288(w195) -> ()
    }
    frame Enabled {
    }
  }
  n81 = xnode "VI-Defined Memory"() -> ("Memory Out"=w8:refnum<k21>)
  n82 = xnode "VI-Defined Memory"() -> ("Memory Out"=w6:refnum<k21>)
  n83 = xnode "VI-Defined Memory"() -> ("Memory Out"=w5:refnum<k21>)
  n84 = node-c288() -> (w30:T23)  [unwired: 1 in]
  n85 = node-c288() -> (w28:T23)  [unwired: 1 in]
  n86 = node-c288() -> (w14:T23)  [unwired: 1 in]
  n87 = node-c288() -> (w26:T23)  [unwired: 1 in]
  n88 = node-c288() -> (w22:T23)  [unwired: 1 in]
  n89 = node-c288() -> (w20:T23)  [unwired: 1 in]
  n90 = timed-loop {
    timing: w30 -> [_]
    timing-out: [_] -> w29
    tunnel: w11 -> [w205]
    tunnel: [w205] -> w10
    stop <- w206 stop-if-true
    n91 = call <vilib>:"Load Analog Replay.vi"("memory"=w205, "load input.<user name>"="load input.VR 1") -> ("done"=w206:bool)  [unwired: 9 in]
  }
  n92 = timed-loop {
    timing: w28 -> [_]
    timing-out: [_] -> w27
    tunnel: w12 -> [w210]
    tunnel: [w210] -> w9
    stop <- w211 stop-if-true
    n93 = call <vilib>:"Load Analog Replay.vi"("memory"=w210, "load input.<user name>"="load input.VR 2") -> ("done"=w211:bool)  [unwired: 9 in]
  }
  n94 = timed-loop {
    timing: w14 -> [_]
    timing-out: [_] -> w13
    tunnel: [w216] -> w1
    stop <- "go.apu 1" stop-if-true
    n95 = call <vilib>:"Create APU Register Bus.vi"("shared settings.<user name>"="shared settings.apu 1") -> ("register bus"=w216:T29)  [unwired: 10 in]
  }
  n96 = disable-structure shown="Disabled" {
    disable-tunnel: w1 -> [w220 _]
    frame Disabled {
      # "Memory should be set to never arbitrate"
      # "Note the naming scheme: \nAll controls / indicators for an analog replay end in the same .<user name>\n<user name> can be anything"
      # "Directional speed sensor memory size should be 1024. It holds that many tooth center positions."
      # "Directional speed sensors should only use high speed digital outputs that can go in a SCTL"
      # "2 Directional Speed Sensors"
      n97 = xnode "VI-Defined Memory"() -> ("Memory Out"=w221:refnum<k21>)
      n98 = xnode "VI-Defined Memory"() -> ("Memory Out"=w223:refnum<k21>)
      n99 = node-c288() -> (w230:T23)  [unwired: 1 in]
      n100 = node-c288() -> (w226:T23)  [unwired: 1 in]
      n101 = timed-loop {
        timing: w230 -> [_]
        timing-out: [_] -> w229
        tunnel: w221 -> [w254]
        tunnel: [w253] -> w222
        stop <- w255 stop-if-true
        n102 = call <vilib>:"Load Directional Speed Sensor.vi"("Memory In"=w254, "load input.<user name>"="load input.Dir Speed 1") -> ("done"=w255:bool, "load data"=w253:T30)  [unwired: 8 in]
      }
      n103 = timed-loop {
        timing: w226 -> [_]
        timing-out: [_] -> w225
        tunnel: w223 -> [w233]
        tunnel: [w232] -> w224
        stop <- w234 stop-if-true
        n104 = call <vilib>:"Load Directional Speed Sensor.vi"("Memory In"=w233, "load input.<user name>"="load input.Dir Speed 2") -> ("done"=w234:bool, "load data"=w232:T30)  [unwired: 8 in]
      }
      n105 = node-c288(w229) -> ()
      n106 = node-c288(w225) -> ()
      n107 = node-c288() -> (w228:T23)  [unwired: 1 in]
      n108 = timed-loop {
        tunnel: w220 -> [w241]
        timing: w228 -> [_]
        timing-out: [_] -> w227
        tunnel: w222 -> [w240]
        tunnel: w224 -> [w239]
        stop <- _ stop-if-true
        # "5V"
        # "See VI context help for a description of controls"
        n109 = call <vilib>:"Directional Speed Sensor.vi"("load data"=w240, "settings.<user name>"="settings.Dir Speed 1", "register bus"=w241, "input.<user name>"="input.Dir Speed 1") -> ("digial output"=w244:bool)  [unwired: 7 in]
        n110 = call <vilib>:"Directional Speed Sensor.vi"("load data"=w239, "settings.<user name>"="settings.Dir Speed 2", "register bus"=w241, "input.<user name>"="input.Dir Speed 2") -> ("digial output"=w245:bool)  [unwired: 7 in]
        n111 = xnode "FPGA I/O Node"("Directional Speed 1"=w244, "Directional Speed 2"=w245) -> ()  [unwired: 2 in, 2 out]
      }
      n112 = node-c288(w227) -> ()
    }
    frame Enabled {
    }
  }
  n113 = timed-loop {
    timing: w26 -> [_]
    timing-out: [_] -> w25
    tunnel: w8 -> [w262]
    tunnel: [w261] -> w7
    stop <- w263 stop-if-true
    n114 = call <vilib>:"Load Digital Pattern Generation.vi"("memory"=w262, "load input.<user name>"="load input.Crank") -> ("done"=w263:bool, "load data"=w261:T28)  [unwired: 8 in]
  }
  n115 = timed-loop {
    timing: w22 -> [_]
    timing-out: [_] -> w21
    tunnel: w6 -> [w268]
    tunnel: [w267] -> w2
    stop <- w269 stop-if-true
    n116 = call <vilib>:"Load Digital Pattern Generation.vi"("memory"=w268, "load input.<user name>"="load input.Cam 1") -> ("done"=w269:bool, "load data"=w267:T28)  [unwired: 8 in]
  }
  n117 = timed-loop {
    timing: w20 -> [_]
    timing-out: [_] -> w19
    tunnel: w5 -> [w274]
    tunnel: [w273] -> w3
    stop <- w275 stop-if-true
    n118 = call <vilib>:"Load Digital Pattern Generation.vi"("memory"=w274, "load input.<user name>"="load input.Cam 2") -> ("done"=w275:bool, "load data"=w273:T28)  [unwired: 8 in]
  }
  n119 = node-c288(w13) -> ()
  n120 = node-c288(w27) -> ()
  n121 = node-c288(w29) -> ()
  n122 = node-c288(w25) -> ()
  n123 = node-c288(w21) -> ()
  n124 = node-c288(w19) -> ()
  n125 = node-c288() -> (w32:T23)  [unwired: 1 in]
  n126 = timed-loop {
    timing: w32 -> [_]
    timing-out: [_] -> w31
    tunnel: w1 -> [w278]
    stop <- _ stop-if-true
    # "See VI context help for a description of controls and indicators"
    n127 = call <vilib>:"Angle Processing Unit.vi"("settings.<user name>"="settings.apu 1", "register bus"=w278, "input.<user name>"="input.apu 1") -> ("output.<user name>"=→"output.apu 1":T4)  [unwired: 8 in]
  }
  n128 = while {
    tunnel: w10 -> [w295]
    tunnel: w1 -> [w284]
    tunnel: w9 -> [w292]
    stop <- FALSE stop-if-true
    # "See VI context help for a description of controls"
    n129 = call <vilib>:"Analog Replay.vi"("shift"=i8 -2, "memory"=w295, "settings.<user name>"="settings.VR 1", "register bus"=w284, "input.<user name>"="input.VR 1") -> ("analog value"=w288:i16)  [unwired: 6 in]
    n130 = call <vilib>:"Analog Replay.vi"("shift"=i8 -2, "memory"=w292, "settings.<user name>"="settings.VR 2", "register bus"=w284, "input.<user name>"="input.VR 2") -> ("analog value"=w287:i16)  [unwired: 6 in]
    n131 = xnode "FPGA I/O Node"("VR 1"=w288, "VR 2"=w287) -> ()  [unwired: 2 in, 2 out]
  }
  n132 = node-c288() -> (w24:T23)  [unwired: 1 in]
  n133 = while {
    tunnel: w1 -> [w297]
    stop <- FALSE stop-if-true
    # "Note: When using C series analog outputs, make sure all outputs to the same module are written with the same IO node to avoid arbitration. Not neccesary for R series."
    n134 = disable-structure shown="Disabled" {
      disable-tunnel: w297 -> [w330 _]
      disable-tunnel: [w327 _] -> w296
      frame Disabled {
        n135 = call <vilib>:"Cylinder Trigger.vi"("settings.<user name>"="settings.Knock 2.Cylinder 1", "register bus"=w330, "input.<user name>"="input.Knock 2.Cylinder 1") -> ("triggered knock data"=w335:T31)  [unwired: 8 in]
        n136 = call <vilib>:"Cylinder Trigger.vi"("settings.<user name>"="settings.Knock 2.Cylinder 2", "register bus"=w330, "input.<user name>"="input.Knock 2.Cylinder 2") -> ("triggered knock data"=w336:T31)  [unwired: 8 in]
        n137 = call <vilib>:"Cylinder Trigger.vi"("settings.<user name>"="settings.Knock 2.Cylinder 3", "register bus"=w330, "input.<user name>"="input.Knock 2.Cylinder 3") -> ("triggered knock data"=w337:T31)  [unwired: 8 in]
        n138 = call <vilib>:"Cylinder Trigger.vi"("settings.<user name>"="settings.Knock 2.Cylinder 5", "register bus"=w330, "input.<user name>"="input.Knock 2.Cylinder 5") -> ("triggered knock data"=w354:T31)  [unwired: 8 in]
        n139 = call <vilib>:"Cylinder Trigger.vi"("settings.<user name>"="settings.Knock 2.Cylinder 7", "register bus"=w330, "input.<user name>"="input.Knock 2.Cylinder 7") -> ("triggered knock data"=w329:T31)  [unwired: 8 in]
        n140 = call <vilib>:"Cylinder Trigger.vi"("settings.<user name>"="settings.Knock 2.Cylinder 4", "register bus"=w330, "input.<user name>"="input.Knock 2.Cylinder 4") -> ("triggered knock data"=w338:T31)  [unwired: 8 in]
        n141 = call <vilib>:"Cylinder Trigger.vi"("settings.<user name>"="settings.Knock 2.Cylinder 6", "register bus"=w330, "input.<user name>"="input.Knock 2.Cylinder 6") -> ("triggered knock data"=w355:T31)  [unwired: 8 in]
        n142 = call <vilib>:"Cylinder Trigger.vi"("settings.<user name>"="settings.Knock 2.Cylinder 8", "register bus"=w330, "input.<user name>"="input.Knock 2.Cylinder 8") -> ("triggered knock data"=w328:T31)  [unwired: 8 in]
        n143 = Build Array(w335, w336, w337, w338, w354, w355, w329, w328) -> (w339:T31[])
        n144 = call <vilib>:"Generate Signal.vi"("settings.<user name>"="settings.Knock 2", "register bus"=w330, "triggered knock data"=w339, "input.<user name>"="input.Knock 2") -> ("knock signal"=w327:i16)  [unwired: 7 in]
      }
      frame Enabled {
        # "2nd knock is disabled\nenable if needed"
      }
    }
    n145 = call <vilib>:"Cylinder Trigger.vi"("settings.<user name>"="settings.Knock 1.Cylinder 1", "register bus"=w297, "input.<user name>"="input.Knock 1.Cylinder 1") -> ("triggered knock data"=w326:T31)  [unwired: 8 in]
    n146 = call <vilib>:"Cylinder Trigger.vi"("settings.<user name>"="settings.Knock 1.Cylinder 2", "register bus"=w297, "input.<user name>"="input.Knock 1.Cylinder 2") -> ("triggered knock data"=w325:T31)  [unwired: 8 in]
    n147 = call <vilib>:"Cylinder Trigger.vi"("settings.<user name>"="settings.Knock 1.Cylinder 3", "register bus"=w297, "input.<user name>"="input.Knock 1.Cylinder 3") -> ("triggered knock data"=w324:T31)  [unwired: 8 in]
    n148 = call <vilib>:"Cylinder Trigger.vi"("settings.<user name>"="settings.Knock 1.Cylinder 5", "register bus"=w297, "input.<user name>"="input.Knock 1.Cylinder 5") -> ("triggered knock data"=w305:T31)  [unwired: 8 in]
    n149 = call <vilib>:"Cylinder Trigger.vi"("settings.<user name>"="settings.Knock 1.Cylinder 4", "register bus"=w297, "input.<user name>"="input.Knock 1.Cylinder 4") -> ("triggered knock data"=w323:T31)  [unwired: 8 in]
    n150 = call <vilib>:"Cylinder Trigger.vi"("settings.<user name>"="settings.Knock 1.Cylinder 6", "register bus"=w297, "input.<user name>"="input.Knock 1.Cylinder 6") -> ("triggered knock data"=w304:T31)  [unwired: 8 in]
    n151 = call <vilib>:"Cylinder Trigger.vi"("settings.<user name>"="settings.Knock 1.Cylinder 7", "register bus"=w297, "input.<user name>"="input.Knock 1.Cylinder 7") -> ("triggered knock data"=w299:T31)  [unwired: 8 in]
    n152 = call <vilib>:"Cylinder Trigger.vi"("settings.<user name>"="settings.Knock 1.Cylinder 8", "register bus"=w297, "input.<user name>"="input.Knock 1.Cylinder 8") -> ("triggered knock data"=w298:T31)  [unwired: 8 in]
    n153 = Build Array(w326, w325, w324, w323, w305, w304, w299, w298) -> (w322:T31[])
    n154 = call <vilib>:"Generate Signal.vi"("settings.<user name>"="settings.Knock 1", "register bus"=w297, "triggered knock data"=w322, "input.<user name>"="input.Knock 1") -> ("knock signal"=w310:i16)  [unwired: 7 in]
    n155 = disable-structure shown="Enabled" {
      disable-tunnel: w310 -> [w357 w358]
      disable-tunnel: w296 -> [w356 _]
      frame Disabled {
        n156 = xnode ("FPGA I/O Node")("Knock 1"=w357, "Connector0/AO3"=w356) -> ()  [unwired: 2 in, 2 out]
      }
      frame Enabled {
        # "2nd knock is disabled\nenable if needed"
        n157 = xnode ("FPGA I/O Node")("Knock 1"=w358) -> ()  [unwired: 1 in, 1 out]
      }
    }
  }
  n158 = timed-loop {
    tunnel: w1 -> [w367]
    timing: w24 -> [_]
    timing-out: [_] -> w23
    tunnel: w7 -> [w366]
    tunnel: w2 -> [w365]
    tunnel: w3 -> [w364]
    tunnel: w4 -> [w363]
    stop <- _ stop-if-true
    # "5V"
    # "See VI context help for a description of controls"
    n159 = disable-structure shown="Disabled" {
      disable-tunnel: w367 -> [w376 _]
      disable-tunnel: w363 -> [w375 _]
      disable-tunnel: [w374 _] -> w359
      frame Disabled {
        n160 = call <vilib>:"Digital Pattern Generation.vi"("load data"=w375, "settings.<user name>"="settings.Aux Pattern", "register bus"=w376, "input.<user name>"="input.Aux Pattern") -> ("digial output"=w374:bool)  [unwired: 7 in]
      }
      frame Enabled {
      }
    }
    n161 = call <vilib>:"Digital Pattern Generation.vi"("load data"=w366, "settings.<user name>"="settings.Crank", "register bus"=w367, "input.<user name>"="input.Crank") -> ("digial output"=w362:bool)  [unwired: 7 in]
    n162 = call <vilib>:"Digital Pattern Generation.vi"("load data"=w365, "settings.<user name>"="settings.Cam 1", "register bus"=w367, "input.<user name>"="input.Cam 1") -> ("digial output"=w361:bool)  [unwired: 7 in]
    n163 = call <vilib>:"Digital Pattern Generation.vi"("load data"=w364, "settings.<user name>"="settings.Cam 2", "register bus"=w367, "input.<user name>"="input.Cam 2") -> ("digial output"=w360:bool)  [unwired: 7 in]
    n164 = xnode "FPGA I/O Node"("Crank"=w362, "Cam 1"=w361, "Cam 2"=w360, "Aux Pattern"=w359) -> ()  [unwired: 4 in, 4 out]
  }
  n165 = node-c288(w31) -> ()
  n166 = node-c288(w23) -> ()
  n167 = node-c288() -> (w18:T23)  [unwired: 1 in]
  n168 = node-c288() -> (w16:T23)  [unwired: 1 in]
  n169 = timed-loop {
    timing: w18 -> [_]
    timing-out: [_] -> w17
    tunnel: w1 -> [w398]
    stop <- _ stop-if-true
    # "See VI context help for a description of controls and indicators"
    n170 = xnode "FPGA I/O Node"() -> ("Spark 1"=w397:bool, "Spark 2"=w395:bool, "Spark 3"=w392:bool, "Spark 4"=w390:bool, "Spark 5"=w388:bool, "Spark 6"=w386:bool, "Spark 7"=w384:bool, "Spark 8"=w382:bool)  [unwired: 8 in, 8 out]
    n171 = call "Digital Filter.vi"("Tics to Filter"="Spark Tics to Filter", "Input Signal"=w395) -> ("Output Filtered Signal"=w394:bool)  [unwired: 9 in]
    n172 = call "Digital Filter.vi"("Tics to Filter"="Spark Tics to Filter", "Input Signal"=w392) -> ("Output Filtered Signal"=w393:bool)  [unwired: 9 in]
    n173 = call "Digital Filter.vi"("Tics to Filter"="Spark Tics to Filter", "Input Signal"=w390) -> ("Output Filtered Signal"=w391:bool)  [unwired: 9 in]
    n174 = call "Digital Filter.vi"("Tics to Filter"="Spark Tics to Filter", "Input Signal"=w388) -> ("Output Filtered Signal"=w389:bool)  [unwired: 9 in]
    n175 = call "Digital Filter.vi"("Tics to Filter"="Spark Tics to Filter", "Input Signal"=w386) -> ("Output Filtered Signal"=w387:bool)  [unwired: 9 in]
    n176 = call "Digital Filter.vi"("Tics to Filter"="Spark Tics to Filter", "Input Signal"=w384) -> ("Output Filtered Signal"=w385:bool)  [unwired: 9 in]
    n177 = call "Digital Filter.vi"("Tics to Filter"="Spark Tics to Filter", "Input Signal"=w382) -> ("Output Filtered Signal"=w383:bool)  [unwired: 9 in]
    n178 = call "Digital Filter.vi"("Tics to Filter"="Spark Tics to Filter", "Input Signal"=w397) -> ("Output Filtered Signal"=w396:bool)  [unwired: 9 in]
    n179 = call-poly <vilib>:"Measure Events.vi"("settings.<user name>"="settings.Event Spark 1", "register bus"=w398, "event"=w396) -> ("measured data"=w432:T33, "status.<user name>"=→"status.Event Spark 1":T7)  [unwired: 7 in]
    n180 = call-poly <vilib>:"Measure Events.vi"("settings.<user name>"="settings.Event Spark 2", "register bus"=w398, "event"=w394) -> ("measured data"=w425:T33, "status.<user name>"=→"status.Event Spark 2":T7)  [unwired: 7 in]
    n181 = call-poly <vilib>:"Measure Events.vi"("settings.<user name>"="settings.Event Spark 3", "register bus"=w398, "event"=w393) -> ("measured data"=w424:T33, "status.<user name>"=→"status.Event Spark 3":T7)  [unwired: 7 in]
    n182 = call-poly <vilib>:"Measure Events.vi"("settings.<user name>"="settings.Event Spark 4", "register bus"=w398, "event"=w391) -> ("measured data"=w423:T33, "status.<user name>"=→"status.Event Spark 4":T7)  [unwired: 7 in]
    n183 = call-poly <vilib>:"Measure Events.vi"("settings.<user name>"="settings.Event Spark 5", "register bus"=w398, "event"=w389) -> ("measured data"=w422:T33, "status.<user name>"=→"status.Event Spark 5":T7)  [unwired: 7 in]
    n184 = call-poly <vilib>:"Measure Events.vi"("settings.<user name>"="settings.Event Spark 6", "register bus"=w398, "event"=w387) -> ("measured data"=w421:T33, "status.<user name>"=→"status.Event Spark 6":T7)  [unwired: 7 in]
    n185 = call-poly <vilib>:"Measure Events.vi"("settings.<user name>"="settings.Event Spark 7", "register bus"=w398, "event"=w385) -> ("measured data"=w406:T33, "status.<user name>"=→"status.Event Spark 7":T7)  [unwired: 7 in]
    n186 = call-poly <vilib>:"Measure Events.vi"("settings.<user name>"="settings.Event Spark 8", "register bus"=w398, "event"=w383) -> ("measured data"=w401:T33, "status.<user name>"=→"status.Event Spark 8":T7)  [unwired: 7 in]
    n187 = call <vilib>:"Capture Event.vi"("event # to capture"=T32 1 ("Settings.spark 1 shot 1"), "measured data"=w432) -> ("capture.<user name>"=→"capture.Event Spark 1.Event 1":T9)  [unwired: 9 in]
    n188 = call <vilib>:"Capture Event.vi"("event # to capture"=T32 1 ("Settings.spark 2 shot 1"), "measured data"=w425) -> ("capture.<user name>"=→"capture.Event Spark 2.Event 1":T9)  [unwired: 9 in]
    n189 = call <vilib>:"Capture Event.vi"("event # to capture"=T32 1 ("Settings.spark 3 shot 1"), "measured data"=w424) -> ("capture.<user name>"=→"capture.Event Spark 3.Event 1":T9)  [unwired: 9 in]
    n190 = call <vilib>:"Capture Event.vi"("event # to capture"=T32 1 ("Settings.spark 4 shot 1"), "measured data"=w423) -> ("capture.<user name>"=→"capture.Event Spark 4.Event 1":T9)  [unwired: 9 in]
    n191 = call <vilib>:"Capture Event.vi"("event # to capture"=T32 1 ("Settings.spark 5 shot 1"), "measured data"=w422) -> ("capture.<user name>"=→"capture.Event Spark 5.Event 1":T9)  [unwired: 9 in]
    n192 = call <vilib>:"Capture Event.vi"("event # to capture"=T32 1 ("Settings.spark 6 shot 1"), "measured data"=w421) -> ("capture.<user name>"=→"capture.Event Spark 6.Event 1":T9)  [unwired: 9 in]
    n193 = call <vilib>:"Capture Event.vi"("event # to capture"=T32 1 ("Settings.spark 6 shot 1"), "measured data"=w406) -> ("capture.<user name>"=→"capture.Event Spark 7.Event 1":T9)  [unwired: 9 in]
    n194 = call <vilib>:"Capture Event.vi"("event # to capture"=T32 1 ("Settings.spark 6 shot 1"), "measured data"=w401) -> ("capture.<user name>"=→"capture.Event Spark 8.Event 1":T9)  [unwired: 9 in]
  }
  n195 = timed-loop {
    timing: w16 -> [_]
    timing-out: [_] -> w15
    tunnel: w1 -> [w441]
    stop <- _ stop-if-true
    # "See VI context help for a description of controls and indicators"
    n196 = xnode "FPGA I/O Node"() -> ("Injector 1"=w558:bool, "Injector 2"=w443:bool, "Injector 3"=w444:bool, "Injector 4"=w445:bool, "Injector 5"=w446:bool, "Injector 6"=w447:bool, "Injector 7"=w448:bool, "Injector 8"=w449:bool)  [unwired: 8 in, 8 out]
    n197 = call "Digital Filter.vi"("Tics to Filter"="Inj Tics to Filter", "Input Signal"=w558) -> ("Output Filtered Signal"=w557:bool)  [unwired: 9 in]
    n198 = call "Digital Filter.vi"("Tics to Filter"="Inj Tics to Filter", "Input Signal"=w443) -> ("Output Filtered Signal"=w538:bool)  [unwired: 9 in]
    n199 = call "Digital Filter.vi"("Tics to Filter"="Inj Tics to Filter", "Input Signal"=w444) -> ("Output Filtered Signal"=w529:bool)  [unwired: 9 in]
    n200 = call "Digital Filter.vi"("Tics to Filter"="Inj Tics to Filter", "Input Signal"=w445) -> ("Output Filtered Signal"=w515:bool)  [unwired: 9 in]
    n201 = call "Digital Filter.vi"("Tics to Filter"="Inj Tics to Filter", "Input Signal"=w446) -> ("Output Filtered Signal"=w501:bool)  [unwired: 9 in]
    n202 = call "Digital Filter.vi"("Tics to Filter"="Inj Tics to Filter", "Input Signal"=w447) -> ("Output Filtered Signal"=w482:bool)  [unwired: 9 in]
    n203 = call "Digital Filter.vi"("Tics to Filter"="Inj Tics to Filter", "Input Signal"=w448) -> ("Output Filtered Signal"=w473:bool)  [unwired: 9 in]
    n204 = call "Digital Filter.vi"("Tics to Filter"="Inj Tics to Filter", "Input Signal"=w449) -> ("Output Filtered Signal"=w454:bool)  [unwired: 9 in]
    n205 = call-poly <vilib>:"Measure Events.vi"("settings.<user name>"="settings.Event Inj 1", "register bus"=w441, "event"=w557) -> ("measured data"=w548:T33, "status.<user name>"=→"status.Event Inj 1":T7)  [unwired: 7 in]
    n206 = call-poly <vilib>:"Measure Events.vi"("settings.<user name>"="settings.Event Inj 2", "register bus"=w441, "event"=w538) -> ("measured data"=w547:T33, "status.<user name>"=→"status.Event Inj 2":T7)  [unwired: 7 in]
    n207 = call-poly <vilib>:"Measure Events.vi"("settings.<user name>"="settings.Event Inj 3", "register bus"=w441, "event"=w529) -> ("measured data"=w520:T33, "status.<user name>"=→"status.Event Inj 3":T7)  [unwired: 7 in]
    n208 = call-poly <vilib>:"Measure Events.vi"("settings.<user name>"="settings.Event Inj 4", "register bus"=w441, "event"=w515) -> ("measured data"=w506:T33, "status.<user name>"=→"status.Event Inj 4":T7)  [unwired: 7 in]
    n209 = call-poly <vilib>:"Measure Events.vi"("settings.<user name>"="settings.Event Inj 5", "register bus"=w441, "event"=w501) -> ("measured data"=w492:T33, "status.<user name>"=→"status.Event Inj 5":T7)  [unwired: 7 in]
    n210 = call-poly <vilib>:"Measure Events.vi"("settings.<user name>"="settings.Event Inj 6", "register bus"=w441, "event"=w482) -> ("measured data"=w491:T33, "status.<user name>"=→"status.Event Inj 6":T7)  [unwired: 7 in]
    n211 = call-poly <vilib>:"Measure Events.vi"("settings.<user name>"="settings.Event Inj 7", "register bus"=w441, "event"=w473) -> ("measured data"=w464:T33, "status.<user name>"=→"status.Event Inj 7":T7)  [unwired: 7 in]
    n212 = call-poly <vilib>:"Measure Events.vi"("settings.<user name>"="settings.Event Inj 8", "register bus"=w441, "event"=w454) -> ("measured data"=w463:T33, "status.<user name>"=→"status.Event Inj 8":T7)  [unwired: 7 in]
    n213 = call <vilib>:"Capture Event.vi"("event # to capture"=T32 1 ("Settings.spark 1 shot 1"), "measured data"=w548) -> ("capture.<user name>"=→"capture.Event Inj 1.Event 1":T9)  [unwired: 9 in]
    n214 = call <vilib>:"Capture Event.vi"("event # to capture"=T32 2 ("Settings.spark 1 shot 1"), "measured data"=w548) -> ("capture.<user name>"=→"capture.Event Inj 1.Event 2":T9)  [unwired: 9 in]
    n215 = call <vilib>:"Capture Event.vi"("event # to capture"=T32 3 ("Settings.spark 1 shot 1"), "measured data"=w548) -> ("capture.<user name>"=→"capture.Event Inj 1.Event 3":T9)  [unwired: 9 in]
    n216 = call <vilib>:"Capture Event.vi"("event # to capture"=T32 4 ("Settings.spark 1 shot 1"), "measured data"=w548) -> ("capture.<user name>"=→"capture.Event Inj 1.Event 4":T9)  [unwired: 9 in]
    n217 = call <vilib>:"Capture Event.vi"("event # to capture"=T32 5 ("Settings.spark 1 shot 1"), "measured data"=w548) -> ("capture.<user name>"=→"capture.Event Inj 1.Event 5":T9)  [unwired: 9 in]
    n218 = call <vilib>:"Capture Event.vi"("event # to capture"=T32 1 ("Settings.spark 1 shot 1"), "measured data"=w547) -> ("capture.<user name>"=→"capture.Event Inj 2.Event 1":T9)  [unwired: 9 in]
    n219 = call <vilib>:"Capture Event.vi"("event # to capture"=T32 2 ("Settings.spark 1 shot 1"), "measured data"=w547) -> ("capture.<user name>"=→"capture.Event Inj 2.Event 2":T9)  [unwired: 9 in]
    n220 = call <vilib>:"Capture Event.vi"("event # to capture"=T32 3 ("Settings.spark 1 shot 1"), "measured data"=w547) -> ("capture.<user name>"=→"capture.Event Inj 2.Event 3":T9)  [unwired: 9 in]
    n221 = call <vilib>:"Capture Event.vi"("event # to capture"=T32 4 ("Settings.spark 1 shot 1"), "measured data"=w547) -> ("capture.<user name>"=→"capture.Event Inj 2.Event 4":T9)  [unwired: 9 in]
    n222 = call <vilib>:"Capture Event.vi"("event # to capture"=T32 5 ("Settings.spark 1 shot 1"), "measured data"=w547) -> ("capture.<user name>"=→"capture.Event Inj 2.Event 5":T9)  [unwired: 9 in]
    n223 = call <vilib>:"Capture Event.vi"("event # to capture"=T32 1 ("Settings.spark 1 shot 1"), "measured data"=w520) -> ("capture.<user name>"=→"capture.Event Inj 3.Event 1":T9)  [unwired: 9 in]
    n224 = call <vilib>:"Capture Event.vi"("event # to capture"=T32 2 ("Settings.spark 1 shot 1"), "measured data"=w520) -> ("capture.<user name>"=→"capture.Event Inj 3.Event 2":T9)  [unwired: 9 in]
    n225 = call <vilib>:"Capture Event.vi"("event # to capture"=T32 3 ("Settings.spark 1 shot 1"), "measured data"=w520) -> ("capture.<user name>"=→"capture.Event Inj 3.Event 3":T9)  [unwired: 9 in]
    n226 = call <vilib>:"Capture Event.vi"("event # to capture"=T32 4 ("Settings.spark 1 shot 1"), "measured data"=w520) -> ("capture.<user name>"=→"capture.Event Inj 3.Event 4":T9)  [unwired: 9 in]
    n227 = call <vilib>:"Capture Event.vi"("event # to capture"=T32 5 ("Settings.spark 1 shot 1"), "measured data"=w520) -> ("capture.<user name>"=→"capture.Event Inj 3.Event 5":T9)  [unwired: 9 in]
    n228 = call <vilib>:"Capture Event.vi"("event # to capture"=T32 1 ("Settings.spark 1 shot 1"), "measured data"=w506) -> ("capture.<user name>"=→"capture.Event Inj 4.Event 1":T9)  [unwired: 9 in]
    n229 = call <vilib>:"Capture Event.vi"("event # to capture"=T32 2 ("Settings.spark 1 shot 1"), "measured data"=w506) -> ("capture.<user name>"=→"capture.Event Inj 4.Event 2":T9)  [unwired: 9 in]
    n230 = call <vilib>:"Capture Event.vi"("event # to capture"=T32 3 ("Settings.spark 1 shot 1"), "measured data"=w506) -> ("capture.<user name>"=→"capture.Event Inj 4.Event 3":T9)  [unwired: 9 in]
    n231 = call <vilib>:"Capture Event.vi"("event # to capture"=T32 4 ("Settings.spark 1 shot 1"), "measured data"=w506) -> ("capture.<user name>"=→"capture.Event Inj 4.Event 4":T9)  [unwired: 9 in]
    n232 = call <vilib>:"Capture Event.vi"("event # to capture"=T32 5 ("Settings.spark 1 shot 1"), "measured data"=w506) -> ("capture.<user name>"=→"capture.Event Inj 4.Event 5":T9)  [unwired: 9 in]
    n233 = call <vilib>:"Capture Event.vi"("event # to capture"=T32 1 ("Settings.spark 1 shot 1"), "measured data"=w492) -> ("capture.<user name>"=→"capture.Event Inj 5.Event 1":T9)  [unwired: 9 in]
    n234 = call <vilib>:"Capture Event.vi"("event # to capture"=T32 2 ("Settings.spark 1 shot 1"), "measured data"=w492) -> ("capture.<user name>"=→"capture.Event Inj 5.Event 2":T9)  [unwired: 9 in]
    n235 = call <vilib>:"Capture Event.vi"("event # to capture"=T32 3 ("Settings.spark 1 shot 1"), "measured data"=w492) -> ("capture.<user name>"=→"capture.Event Inj 5.Event 3":T9)  [unwired: 9 in]
    n236 = call <vilib>:"Capture Event.vi"("event # to capture"=T32 4 ("Settings.spark 1 shot 1"), "measured data"=w492) -> ("capture.<user name>"=→"capture.Event Inj 5.Event 4":T9)  [unwired: 9 in]
    n237 = call <vilib>:"Capture Event.vi"("event # to capture"=T32 5 ("Settings.spark 1 shot 1"), "measured data"=w492) -> ("capture.<user name>"=→"capture.Event Inj 5.Event 5":T9)  [unwired: 9 in]
    n238 = call <vilib>:"Capture Event.vi"("event # to capture"=T32 1 ("Settings.spark 1 shot 1"), "measured data"=w491) -> ("capture.<user name>"=→"capture.Event Inj 6.Event 1":T9)  [unwired: 9 in]
    n239 = call <vilib>:"Capture Event.vi"("event # to capture"=T32 2 ("Settings.spark 1 shot 1"), "measured data"=w491) -> ("capture.<user name>"=→"capture.Event Inj 6.Event 2":T9)  [unwired: 9 in]
    n240 = call <vilib>:"Capture Event.vi"("event # to capture"=T32 3 ("Settings.spark 1 shot 1"), "measured data"=w491) -> ("capture.<user name>"=→"capture.Event Inj 6.Event 3":T9)  [unwired: 9 in]
    n241 = call <vilib>:"Capture Event.vi"("event # to capture"=T32 4 ("Settings.spark 1 shot 1"), "measured data"=w491) -> ("capture.<user name>"=→"capture.Event Inj 6.Event 4":T9)  [unwired: 9 in]
    n242 = call <vilib>:"Capture Event.vi"("event # to capture"=T32 5 ("Settings.spark 1 shot 1"), "measured data"=w491) -> ("capture.<user name>"=→"capture.Event Inj 6.Event 5":T9)  [unwired: 9 in]
    n243 = call <vilib>:"Capture Event.vi"("event # to capture"=T32 1 ("Settings.spark 1 shot 1"), "measured data"=w464) -> ("capture.<user name>"=→"capture.Event Inj 7.Event 1":T9)  [unwired: 9 in]
    n244 = call <vilib>:"Capture Event.vi"("event # to capture"=T32 2 ("Settings.spark 1 shot 1"), "measured data"=w464) -> ("capture.<user name>"=→"capture.Event Inj 7.Event 2":T9)  [unwired: 9 in]
    n245 = call <vilib>:"Capture Event.vi"("event # to capture"=T32 3 ("Settings.spark 1 shot 1"), "measured data"=w464) -> ("capture.<user name>"=→"capture.Event Inj 7.Event 3":T9)  [unwired: 9 in]
    n246 = call <vilib>:"Capture Event.vi"("event # to capture"=T32 4 ("Settings.spark 1 shot 1"), "measured data"=w464) -> ("capture.<user name>"=→"capture.Event Inj 7.Event 4":T9)  [unwired: 9 in]
    n247 = call <vilib>:"Capture Event.vi"("event # to capture"=T32 5 ("Settings.spark 1 shot 1"), "measured data"=w464) -> ("capture.<user name>"=→"capture.Event Inj 7.Event 5":T9)  [unwired: 9 in]
    n248 = call <vilib>:"Capture Event.vi"("event # to capture"=T32 1 ("Settings.spark 1 shot 1"), "measured data"=w463) -> ("capture.<user name>"=→"capture.Event Inj 8.Event 1":T9)  [unwired: 9 in]
    n249 = call <vilib>:"Capture Event.vi"("event # to capture"=T32 2 ("Settings.spark 1 shot 1"), "measured data"=w463) -> ("capture.<user name>"=→"capture.Event Inj 8.Event 2":T9)  [unwired: 9 in]
    n250 = call <vilib>:"Capture Event.vi"("event # to capture"=T32 3 ("Settings.spark 1 shot 1"), "measured data"=w463) -> ("capture.<user name>"=→"capture.Event Inj 8.Event 3":T9)  [unwired: 9 in]
    n251 = call <vilib>:"Capture Event.vi"("event # to capture"=T32 4 ("Settings.spark 1 shot 1"), "measured data"=w463) -> ("capture.<user name>"=→"capture.Event Inj 8.Event 4":T9)  [unwired: 9 in]
    n252 = call <vilib>:"Capture Event.vi"("event # to capture"=T32 5 ("Settings.spark 1 shot 1"), "measured data"=w463) -> ("capture.<user name>"=→"capture.Event Inj 8.Event 5":T9)  [unwired: 9 in]
  }
  n253 = node-c288(w17) -> ()
  n254 = node-c288(w15) -> ()
